vi "UpdateTestingResults.vi"(8 "Variant":string, 9 "SerialNumber":string, 10 "NewData":u8[](array[numeric]), 11 "index (row)":i32) -> ()   [LabVIEW 2025]
uses:
  <vilib>/Utility/file.llb/Read Delimited Spreadsheet (I64).vi
  <vilib>/Utility/file.llb/Write Delimited Spreadsheet (I64).vi
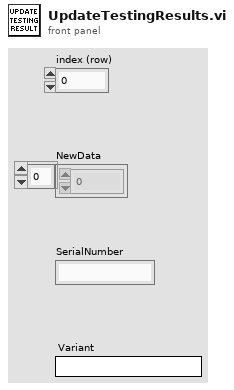
[diagram p1: front panel]
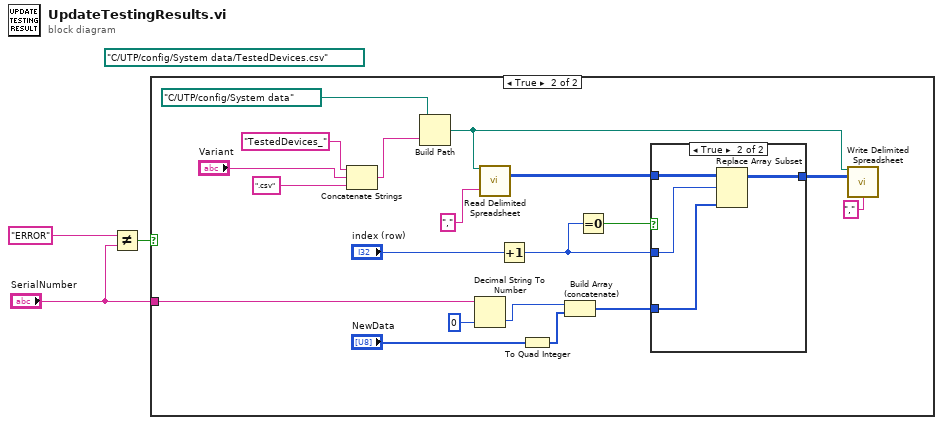
[diagram p0: block diagram]
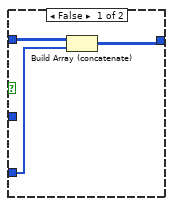
[diagram p3: hidden frame]
diagram:
  (unwired) path "C:/UTP/config/System data/TestedDevices.csv" ("file path (dialog if empty)")
  n1 = Not Equal?(x="ERROR", y="SerialNumber") -> (x != y?=w2:bool)
  n2 = case shown="True" w2 {
    tunnel: "SerialNumber" -> [_ w18]
    frame False {
    }
    frame True {
      n3 = Concatenate Strings("TestedDevices_" ("string"), "Variant", ".csv" ("string")) -> (w7:string)
      n4 = Build Path(base path=path "C:/UTP/config/System data" ("file path (dialog if empty)"), name or relative path=w7) -> (appended path=w5:path)
      n5 = Decimal String To Number(string=w18, default (0L)=i64 0) -> (number=w16:i64)  [unwired: 1 in, 1 out]
      n6 = call-poly <vilib>:"Read Delimited Spreadsheet.vi"("file path (dialog if empty)"=w5, "delimiter (\\t)"="," ("delimiter (\\t)")) -> ("all rows"=w12:i64[][])  [unwired: 8 in, 5 out]
      n7 = Increment(x="index (row)") -> (x+1=w10:i32)
      n8 = To Quad Integer(1:"NewData") -> (0:w13:i64[])
      n9 = Build Array (concatenate)(w16, w13) -> (w14:i64[])
      n10 = Equal To 0?(x=w10) -> (x = 0?=w11:bool)
      n11 = case shown="True" w11 {
        tunnel: [w24 w29] -> w20
        tunnel: w14 -> [w23 w28]
        tunnel: w12 -> [w25 w27]
        tunnel: w10 -> [_ w26]
        frame False {
          n12 = Build Array (concatenate)(w25, w23) -> (w24:i64[][])
        }
        frame True {
          n13 = Replace Array Subset(array=w27, new element=w28, index (row)=w26) -> (w29:i64[][])  [unwired: 1 in]
        }
      }
      n14 = call-poly <vilib>:"Write Delimited Spreadsheet.vi"("file path (dialog if empty)"=w5, "2D data"=w20, "delimiter (\\t)"="," ("delimiter (\\t)")) -> ()  [unwired: 11 in, 2 out]
    }
  }
